vi "sequence structure record-write.vi"   [LabVIEW 2015]
uses:
  <vilib>/Platform/TimedLoop/XDataNode/timing_clust.ctl
  <vilib>/Platform/TimedLoop/XDataNode/nitl_modes.ctl
  <vilib>/Platform/TimedLoop/XDataNode/wakeup.ctl
  <vilib>/Rock Robotics/WPI/Utilities/WPI_GetSetVariantRefNum.vi
  Robot Global Data.vi
  <vilib>/platform/TimedLoop/XDataNode/XDataNode.xnode
  <vilib>/Platform/TimedLoop/XDataNode/XDNodeRunTimeDep.lvlib
types:
  T1 = typedef "WPI_MotorControlDeviceRef.ctl" = cluster{"DeviceStatus":errorcluster, "Type":T2, "PWM":cluster{"PWM Channel":T3, "DeadBand":T4}, "CAN":cluster{"Device Number":u8, "Control Mode":T5, "Semaphore":T6, "Max Vout":dbl, "TalonSRX Control Mode":T7}, "Invert":bool}
  T2 = typedef "WPI_MotorControlType.ctl" = enum16{"PWM", "CAN", "CANTalonSRX"}
  T3 = typedef "FPGA_DIOPWMChannel.ctl" = enum8{"PWM 0", "PWM 1", "PWM 2", "PWM 3", "PWM 4", "PWM 5", "PWM 6", "PWM 7", "PWM 8", "PWM 9", "PWM MXP 0", "PWM MXP 1", "PWM MXP 2", "PWM MXP 3", "PWM MXP 4", "PWM MXP 5", "PWM MXP 6", "PWM MXP 7", "PWM MXP 8", "PWM MXP 9", "Invalid"}
  T4 = typedef "WPI_PWMDeadband.ctl" = cluster{"Name":string, "maxPositivePwm":i32, "minPositivePwm":i32, "centerPwm":i32, "maxNegativePwm":i32, "minNegativePwm":i32, "angularRange":u16}
  T5 = typedef "WPI_CANJaguar_ControlMode.ctl" = enum8{"Percent VBus", "Current", "Speed", "Position", "Voltage"}
  T6 = typedef "Semaphore RefNum" = refnum<k1>
  T7 = typedef "WPI_CANTalonSRX_APIControlMode.ctl" = enum8{"Percent VBus", "Speed", "Position", "Slave", "Unchanged / Invalid", "Voltage Compensation", "Current", "Motion Profile"}
  T8 = typedef "WPI_JoystickDevRef.ctl" = cluster{"Device":T9}
  T9 = typedef "WPI_JoystickDeviceEnum.ctl" = enum16{"USB 0", "USB 1", "USB 2", "USB 3", "USB 4", "USB 5"}
  T10 = typedef "XDNodeRunTimeDep.lvlib/timing_clust.ctl" = cluster{"Expected End [f-1]":u64, "Actual End [f-1]":u64, "Finished Late? [f-1]":bool, "Expected End [i-1]":u64, "Actual End [i-1]":u64, "Finished Late? [i-1]":bool, "Expected Start [i]":u64, "Actual Start [i]":u64, "Expected Start [f]":u64, "Actual Start [f]":u64, "Source Name":string, "Structure Name":string, "Period":i64, "Deadline":i64, "Offset":i64, "Start":i64, "Priority":i32, "Timeout":i32, "Mode":T11, "Wakeup Reason":T12, "Error":errorcluster, "Source Type":string, "Secondary Source Type":string, "Global End Time":u64, "Global Start Time":u64, "Frame Duration":u64, "Iteration Duration":u64, "Assigned CPU":i32, "I/O Scan Engine Mode":u32}
  T11 = typedef "XDNodeRunTimeDep.lvlib/nitl_modes.ctl" = enum32{"No Change", "Process missed periods, maintain original phase", "Discard missed periods, maintain original phase", "Process missed periods, ignore original phase", "Discard missed periods, ignore original phase"}
  T12 = typedef "XDNodeRunTimeDep.lvlib/wakeup.ctl" = enum32{"Normal", "Aborted", "Asynchronous wakeup", "Timing source error", "Timed loop error", "Timeout"}
  T13 = enum16{"open", "replace", "create", "open or create", "replace or create", "replace or create with confirmation"}
  T14 = cluster{"Record?":bool, "Current File":string, "Run script?":bool, "Stop recording?":bool, "Stop script?":bool}
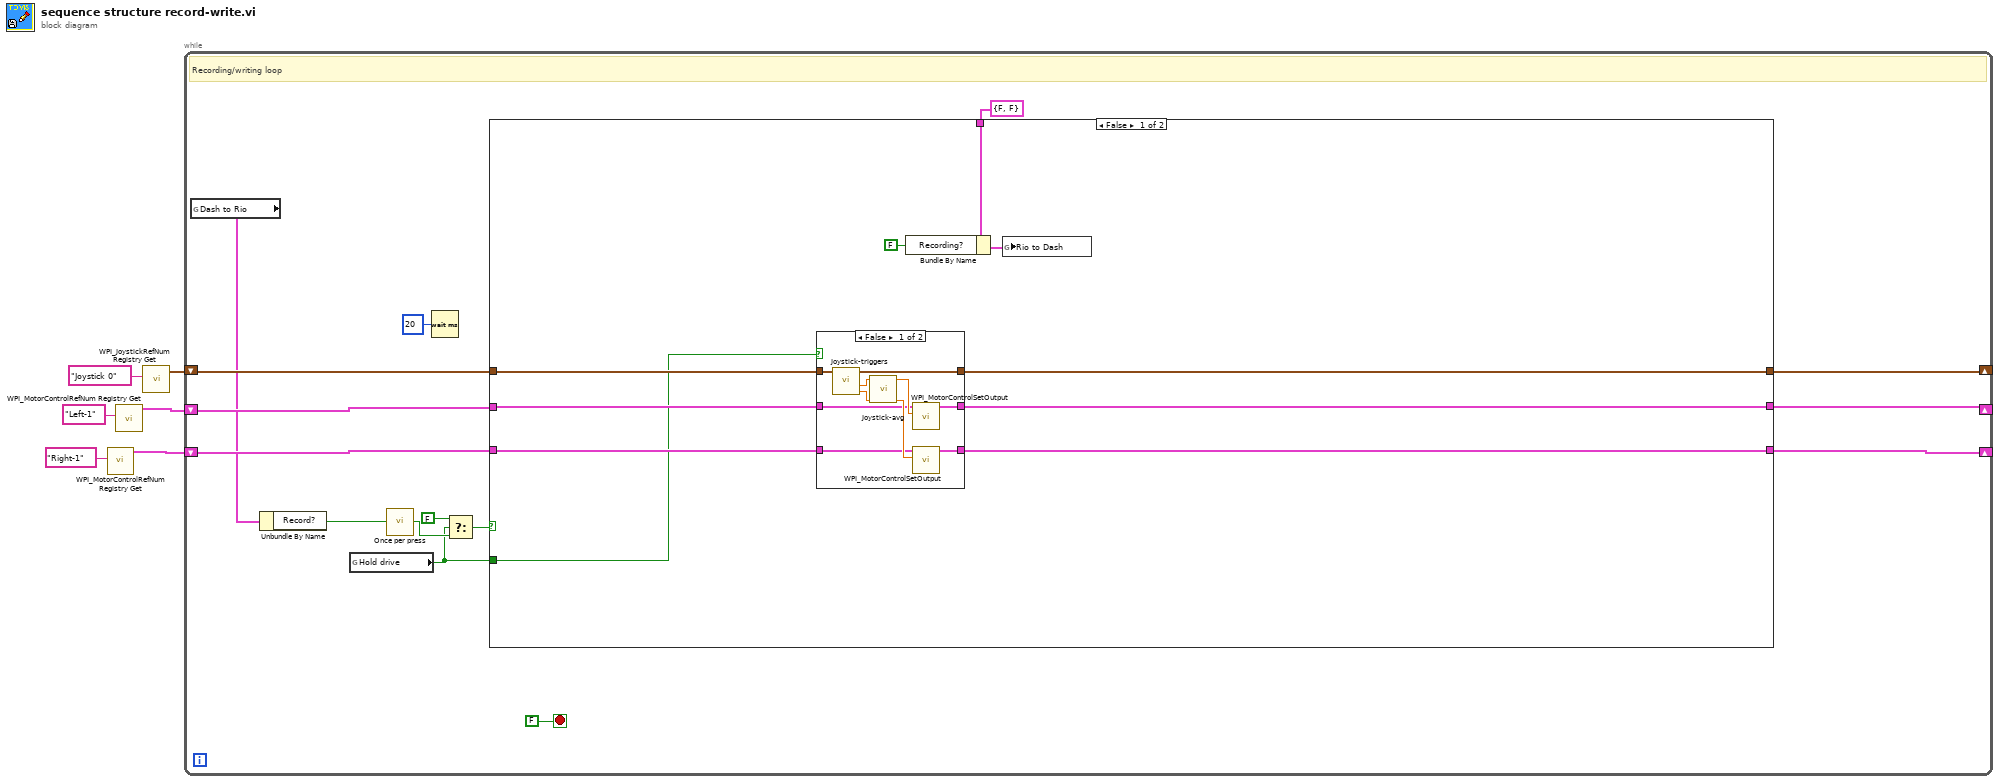
[diagram p0: block diagram]
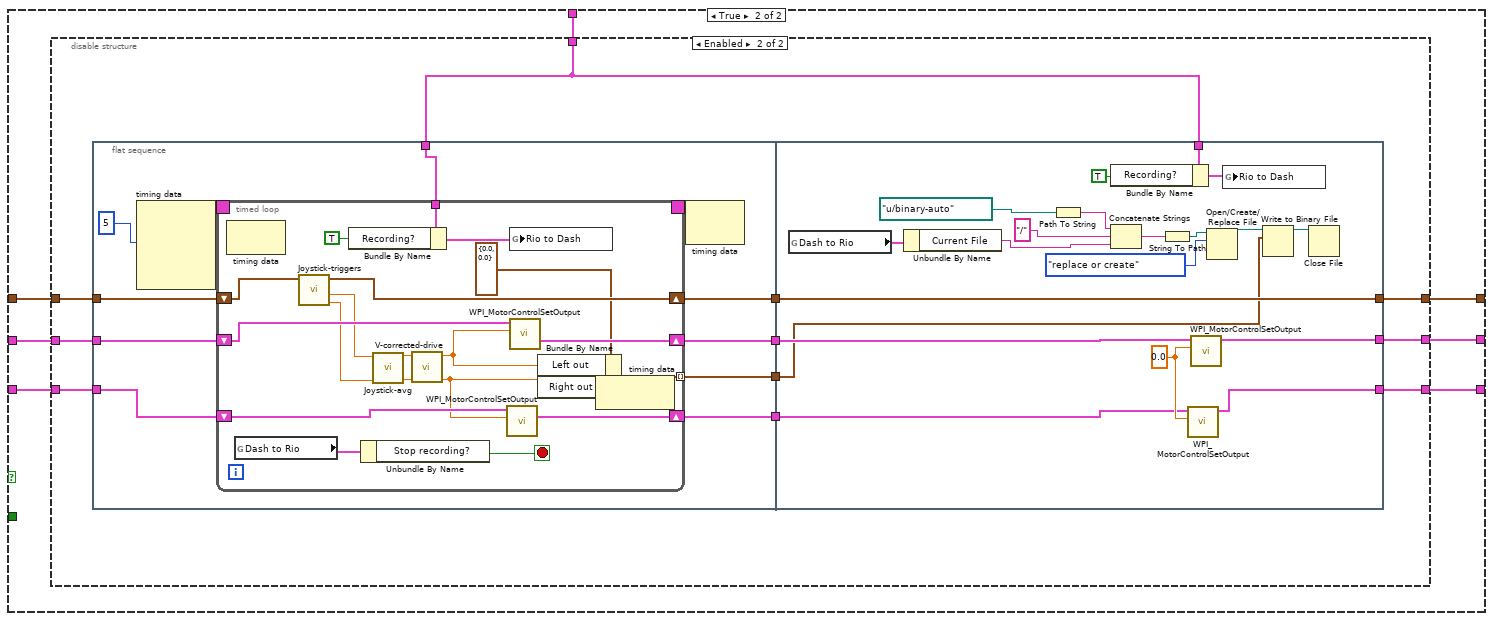
[diagram p3: hidden frame]
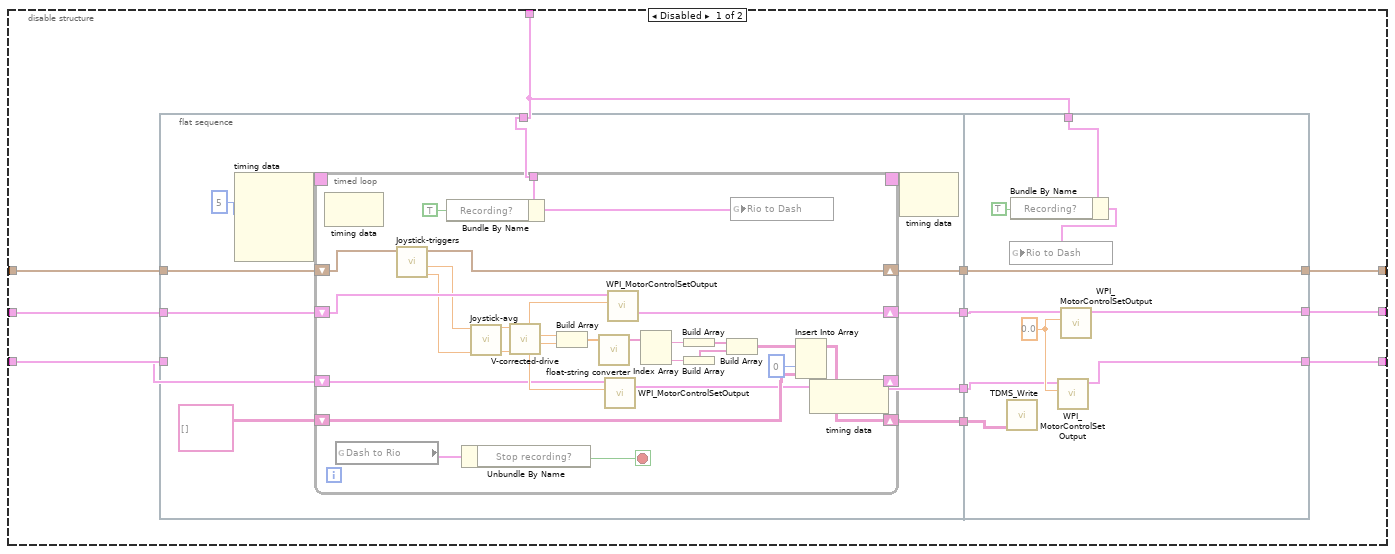
[diagram p4: hidden frame]
diagram:
  n1 = call <vilib>:"WPI_MotorControlRefNum Registry Get.vi"("refnum name"="Right-1") -> ("MotorControlDevRef"=w2:T1)  [unwired: 9 in, 1 out]
  n2 = call <vilib>:"WPI_MotorControlRefNum Registry Get.vi"("refnum name"="Left-1") -> ("MotorControlDevRef"=w1:T1)  [unwired: 9 in, 1 out]
  n3 = call <vilib>:"WPI_JoystickRefNum Registry Get.vi"("refnum name"="Joystick 0") -> ("JoystickDevRef"=w3:T8)  [unwired: 1 in, 9 out]
  n4 = while {
    shift-right: [w15] -> _
    shift-left: w1 -> [w18]
    shift-right: [w14] -> _
    shift-left: w2 -> [w17]
    shift-right: [w16] -> _
    shift-left: w3 -> [w19]
    stop <- FALSE stop-if-true
    # "Recording/writing loop"
    n5 = global read "Robot Global Data.vi" "Dash to Rio"() -> (w8:T14)
    n6 = Unbundle By Name(w8) -> ("Record?"=w9:bool)
    n7 = global read "Robot Global Data.vi" "Hold drive"() -> (w10:bool)
    n8 = call "Once per press.vi"("In"=w9) -> ("Out"=w12:bool)  [unwired: 2 in]
    n9 = Wait (ms)(milliseconds to wait=u32 20) -> ()  [unwired: 1 out]
    n10 = Select(t=FALSE, s=w10, f=w12) -> (s? t:f=w13:bool)
    n11 = case shown="False" w13 {
      tunnel: w19 -> [w31 w51]
      tunnel: w18 -> [w27 w50]
      tunnel: w17 -> [w26 w49]
      tunnel: [w30 w48] -> w16
      tunnel: [w28 w47] -> w15
      tunnel: [w29 w46] -> w14
      tunnel: w10 -> [w25 _]
      tunnel: cluster{"Recording?":bool, "Running?":bool} {"Recording?"=FALSE, "Running?"=FALSE} ("Rio to Dash") -> [w23 w45]
      frame False {
        n12 = case shown="False" w25 {
          tunnel: w31 -> [w39 w44]
          tunnel: [w38 w44] -> w30
          tunnel: [w35 w42] -> w29
          tunnel: [w34 w43] -> w28
          tunnel: w27 -> [w33 w43]
          tunnel: w26 -> [w32 w42]
          frame False {
            n13 = call "Joystick-triggers.vi"("JoystickDevRef"=w39) -> ("Right out"=w40:dbl, "Left out"=w41:dbl, "JoystickDevRef out"=w38:T8)  [unwired: 6 in, 2 out]
            n14 = call "Joystick-avg.vi"("Joystic right axis in"=w40, "Joystic left axis in"=w41) -> ("Right out"=w36:dbl, "Left out"=w37:dbl)  [unwired: 8 in]
            n15 = call <vilib>:"WPI_MotorControlSetOutput.vi"("Output"=w37, "MotorControlDevRef"=w33) -> ("MotorControlDevRef"=w34:T1)  [unwired: 7 in, 2 out]
            n16 = call <vilib>:"WPI_MotorControlSetOutput.vi"("Output"=w36, "MotorControlDevRef"=w32) -> ("MotorControlDevRef"=w35:T1)  [unwired: 7 in, 2 out]
          }
          frame True {
          }
        }
        n17 = Bundle By Name(cluster=w23, "Recording?"=FALSE) -> (w24:cluster{"Recording?":bool, "Running?":bool})
        n18 = global write "Robot Global Data.vi" "Rio to Dash"(w24) -> ()
      }
      frame True {
        n19 = disable-structure shown="Enabled" {
          disable-tunnel: w51 -> [w58 w125]
          disable-tunnel: w50 -> [w57 w124]
          disable-tunnel: w49 -> [w56 w123]
          disable-tunnel: [w55 w122] -> w48
          disable-tunnel: [w54 w121] -> w47
          disable-tunnel: [w53 w120] -> w46
          disable-tunnel: w45 -> [w52 w119]
          frame Disabled {
            n20 = flat-sequence {
              tunnel: [w70] -> w62
              tunnel: w58 -> [w69]
              tunnel: w57 -> [w68]
              tunnel: w56 -> [w67]
              tunnel: [w66] -> w61
              tunnel: [w65] -> w60
              tunnel: [w64] -> w59
              tunnel: w52 -> [w63]
              tunnel: w62 -> [w117]
              tunnel: w61 -> [w115]
              tunnel: w60 -> [w114]
              tunnel: [w113] -> w55
              tunnel: w59 -> [w113]
              tunnel: [w112] -> w54
              tunnel: [w111] -> w53
              tunnel: w52 -> [w110]
              frame #0 {
                n21 = node-c288(i64 5 ("Period")) -> (w74:T10)  [unwired: 3 in]
                n22 = timed-loop {
                  timing: w74 -> [_]
                  timing-out: [_] -> w73
                  shift-right: [w92] -> w70
                  shift-left: string[][] [] -> [w93]
                  shift-right: [w86] -> w65
                  shift-left: w67 -> [w87]
                  shift-right: [w84] -> w66
                  shift-left: w68 -> [w85]
                  shift-right: [w82] -> w64
                  shift-left: w69 -> [w83]
                  tunnel: w63 -> [w75]
                  stop <- w78 stop-if-true
                  n23 = node-c288() -> ()  [unwired: 1 in, 1 out]
                  n24 = global read "Robot Global Data.vi" "Dash to Rio"() -> (w79:T14)
                  n25 = call "Joystick-triggers.vi"("JoystickDevRef"=w83) -> ("Right out"=w80:dbl, "Left out"=w81:dbl, "JoystickDevRef out"=w82:T8)  [unwired: 6 in, 2 out]
                  n26 = Bundle By Name(cluster=w75, "Recording?"=TRUE) -> (w76:cluster{"Recording?":bool, "Running?":bool})
                  n27 = Unbundle By Name(w79) -> ("Stop recording?"=w78:bool)
                  n28 = call "Joystick-avg.vi"("Joystic right axis in"=w80, "Joystic left axis in"=w81) -> ("Right out"=w90:dbl, "Left out"=w91:dbl)  [unwired: 8 in]
                  n29 = call "V-corrected-drive.vi"("R-IN"=w90, "L-IN 2"=w91) -> ("Right out"=w89:dbl, "Left out"=w88:dbl)  [unwired: 8 in]
                  n30 = Build Array(w88, w89) -> (w97:dbl[])
                  n31 = call "float-string converter.vi"("float in"=w97) -> ("float string out"=w96:string[])  [unwired: 3 in, 1 out]
                  n32 = call <vilib>:"WPI_MotorControlSetOutput.vi"("Output"=w89, "MotorControlDevRef"=w87) -> ("MotorControlDevRef"=w86:T1)  [unwired: 7 in, 2 out]
                  n33 = call <vilib>:"WPI_MotorControlSetOutput.vi"("Output"=w88, "MotorControlDevRef"=w85) -> ("MotorControlDevRef"=w84:T1)  [unwired: 7 in, 2 out]
                  n34 = Index Array(array=w96) -> (element #1=w95:string, element #2=w94:string)  [unwired: 2 in]
                  n35 = Build Array(w95) -> (w100:string[])
                  n36 = Build Array(w94) -> (w101:string[])
                  n37 = Build Array(w100, w101) -> (w99:string[][])
                  n38 = global write "Robot Global Data.vi" "Rio to Dash"(w76) -> ()
                  n39 = Insert Into Array(array=w99, index (col)=0 ("disabled index (col)"), new element=w93) -> (w92:string[][])  [unwired: 1 in]
                  n40 = node-c288() -> ()  [unwired: 1 in, 1 out]
                }
                n41 = node-c288(w73) -> ()  [unwired: 1 out]
              }
              frame #1 {
                w116 = 0.0 ("Output")
                n42 = call "TDMS_Write.vi"("2D data array"=w117) -> ()  [unwired: 11 in]
                n43 = Bundle By Name(cluster=w110, "Recording?"=TRUE) -> (w108:cluster{"Recording?":bool, "Running?":bool})
                n44 = global write "Robot Global Data.vi" "Rio to Dash"(w108) -> ()
                n45 = call <vilib>:"WPI_MotorControlSetOutput.vi"("Output"=w116, "MotorControlDevRef"=w114) -> ("MotorControlDevRef"=w111:T1)  [unwired: 7 in, 2 out]
                n46 = call <vilib>:"WPI_MotorControlSetOutput.vi"("Output"=w116, "MotorControlDevRef"=w115) -> ("MotorControlDevRef"=w112:T1)  [unwired: 7 in, 2 out]
              }
            }
          }
          frame Enabled {
            n47 = flat-sequence {
              tunnel: w125 -> [w136]
              tunnel: w124 -> [w135]
              tunnel: w123 -> [w134]
              tunnel: [w133] -> w128
              tunnel: [w132] -> w127
              tunnel: [w131] -> w126
              tunnel: w119 -> [w130]
              tunnel: [w129] -> w118
              tunnel: w128 -> [w183]
              tunnel: w127 -> [w182]
              tunnel: [w181] -> w122
              tunnel: w126 -> [w181]
              tunnel: [w180] -> w121
              tunnel: [w179] -> w120
              tunnel: w119 -> [w178]
              tunnel: w118 -> [w165]
              frame #0 {
                n48 = node-c288(i64 5 ("Period")) -> (w139:T10)  [unwired: 3 in]
                n49 = timed-loop {
                  timing: w139 -> [_]
                  timing-out: [_] -> w138
                  shift-right: [w155] -> w132
                  shift-left: w134 -> [w156]
                  shift-right: [w153] -> w133
                  shift-left: w135 -> [w154]
                  shift-right: [w151] -> w131
                  shift-left: w136 -> [w152]
                  tunnel: w130 -> [w144]
                  tunnel: [w141] -> w129 mode=indexing
                  stop <- w147 stop-if-true
                  n50 = node-c288() -> ()  [unwired: 1 in, 1 out]
                  n51 = global read "Robot Global Data.vi" "Dash to Rio"() -> (w148:T14)
                  n52 = call "Joystick-triggers.vi"("JoystickDevRef"=w152) -> ("Right out"=w149:dbl, "Left out"=w150:dbl, "JoystickDevRef out"=w151:T8)  [unwired: 6 in, 2 out]
                  n53 = Bundle By Name(cluster=w144, "Recording?"=TRUE) -> (w145:cluster{"Recording?":bool, "Running?":bool})
                  n54 = Unbundle By Name(w148) -> ("Stop recording?"=w147:bool)
                  n55 = call "Joystick-avg.vi"("Joystic right axis in"=w149, "Joystic left axis in"=w150) -> ("Right out"=w157:dbl, "Left out"=w158:dbl)  [unwired: 8 in]
                  n56 = call "V-corrected-drive.vi"("R-IN"=w157, "L-IN 2"=w158) -> ("Right out"=w142:dbl, "Left out"=w143:dbl)  [unwired: 8 in]
                  n57 = call <vilib>:"WPI_MotorControlSetOutput.vi"("Output"=w142, "MotorControlDevRef"=w156) -> ("MotorControlDevRef"=w155:T1)  [unwired: 7 in, 2 out]
                  n58 = global write "Robot Global Data.vi" "Rio to Dash"(w145) -> ()
                  n59 = call <vilib>:"WPI_MotorControlSetOutput.vi"("Output"=w143, "MotorControlDevRef"=w154) -> ("MotorControlDevRef"=w153:T1)  [unwired: 7 in, 2 out]
                  n60 = Bundle By Name(cluster=cluster{"Left out":dbl, "Right out":dbl} {"Left out"=0.0, "Right out"=0.0}, "Left out"=w143, "Right out"=w142) -> (w141:cluster{"Left out":dbl, "Right out":dbl})
                  n61 = node-c288() -> ()  [unwired: 1 in, 1 out]
                }
                n62 = node-c288(w138) -> ()  [unwired: 1 out]
              }
              frame #1 {
                w184 = 0.0 ("Output")
                n63 = global read "Robot Global Data.vi" "Dash to Rio"() -> (w169:T14)
                n64 = Unbundle By Name(w169) -> ("Current File"=w170:string)
                n65 = Path To String(path=path "u:/binary-auto" ("file path 3")) -> (string=w166:string)
                n66 = Bundle By Name(cluster=w178, "Recording?"=TRUE) -> (w176:cluster{"Recording?":bool, "Running?":bool})
                n67 = Concatenate Strings(w166, "/" ("TDMS file name"), w170) -> (w168:string)
                n68 = String To Path(string=w168) -> (path=w172:path)
                n69 = call <vilib>:"WPI_MotorControlSetOutput.vi"("Output"=w184, "MotorControlDevRef"=w182) -> ("MotorControlDevRef"=w179:T1)  [unwired: 7 in, 2 out]
                n70 = call <vilib>:"WPI_MotorControlSetOutput.vi"("Output"=w184, "MotorControlDevRef"=w183) -> ("MotorControlDevRef"=w180:T1)  [unwired: 7 in, 2 out]
                n71 = Open/Create/Replace File(file path (use dialog)=w172, operation (0:open)=T13."replace or create") -> (refnum out=w174:refnum<file>)  [unwired: 4 in, 2 out]
                n72 = global write "Robot Global Data.vi" "Rio to Dash"(w176) -> ()
                n73 = Write to Binary File(file (use dialog)=w174, data=w165) -> (refnum out=w175:refnum<file>)  [unwired: 4 in, 2 out]
                n74 = Close File(refnum=w175) -> ()  [unwired: 1 in, 2 out]
              }
            }
          }
        }
      }
    }
  }
